vi "LV to DAT 1D.vi"(4 "append to file? (new file:F)":bool, 6 "wavenames (.Vx, etc)":string[](array[string]), 7 "filename":string, 8 "error in":errorcluster, 9 "Data":dbl[](array[numeric]), 10 "Comments":string, 11 "path":path) -> (0 "error out":errorcluster, 3 "new file path":path)   [LabVIEW 2016, in "LV to ITX.lvclass"]
uses:
  LV to ITX.lvclass
  Typedefs/Filetype--enum.ctl
  <vilib>/Utility/file.llb/Write Delimited Spreadsheet (string).vi
panel:
  out "appended array":string[][](array[string])
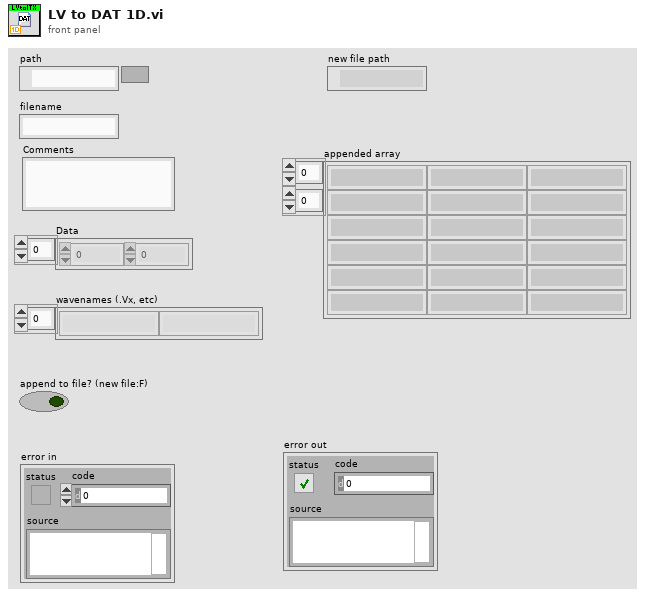
[diagram p1: front panel]
types:
  T1 = typedef "LV to ITX.lvclass/Filetype--enum.ctl" = enum16{"DAT", "ITX", "HDF5", "TDMS", "VI"}
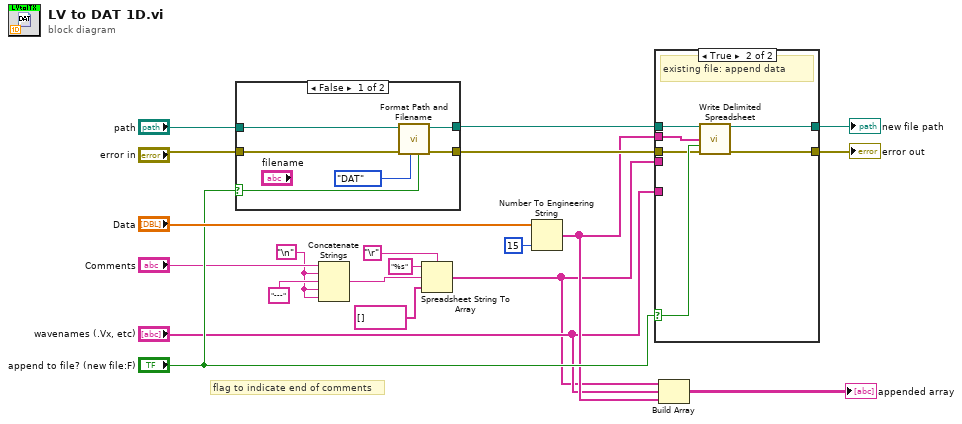
[diagram p0: block diagram]
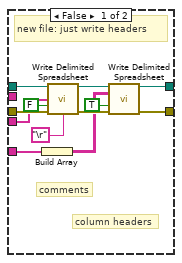
[diagram p3: hidden frame]
diagram:
  w6 = "\n"
  # "flag to indicate end of comments"
  n1 = case shown="False" "append to file? (new file:F)" {
    selector: "append to file? (new file:F)" -> [w22 _]
    tunnel: [w24 w28] -> w20
    tunnel: "path" -> [w25 w28]
    tunnel: "error in" -> [w26 w27]
    tunnel: [w23 w27] -> w14
    frame False {
      n2 = call "Format Path and Filename.vi"("append? (F)"=w22, "Type (TDMS)"=Filetype--enum."DAT", "error in"=w26, "path"=w25) -> ("error out"=w23:errorcluster, "path"=w24:path)  [unwired: 5 in, 1 out]
    }
    frame True {
    }
  }
  n3 = Concatenate Strings("Comments", w6, "---" ("string"), w6, w6) -> (w11:string)
  n4 = Spreadsheet String To Array(delimiter (Tab)="\r", format string="%s", spreadsheet string=w11, array type (2D Dbl)=string[] []) -> (array=w2:string[])
  n5 = Number To Engineering String(2:i16 15 ("precision (6)"), 4:"Data") -> (0:w4:string[])  [unwired: 2 out]
  n6 = case shown="True" "append to file? (new file:F)" {
    selector: "append to file? (new file:F)" -> [_ w45]
    tunnel: w2 -> [w33 _]
    tunnel: [w38 w42] -> w13
    tunnel: w4 -> [_ w44]
    tunnel: w20 -> [w40 w46]
    tunnel: w14 -> [w39 w43]
    tunnel: [w35 w41] -> w12
    tunnel: "wavenames (.Vx, etc)" -> [w32 _]
    frame False {
      # "column headers"
      # "comments"
      # "new file: just write headers"
      n7 = Build Array(w32) -> (w31:string[][])
      n8 = call-poly <vilib>:"Write Delimited Spreadsheet.vi"("file path (dialog if empty)"=w40, "1D data"=w33, "append to file? (new file:F)"=FALSE, "error in (no error)"=w39, "delimiter (\\t)"="\r") -> ("new file path (Not A Path if cancelled)"=w36:path, "error out"=w37:errorcluster)  [unwired: 9 in]
      n9 = call-poly <vilib>:"Write Delimited Spreadsheet.vi"("file path (dialog if empty)"=w36, "2D data"=w31, "append to file? (new file:F)"=TRUE, "error in (no error)"=w37) -> ("new file path (Not A Path if cancelled)"=w38:path, "error out"=w35:errorcluster)  [unwired: 10 in]
    }
    frame True {
      # "existing file: append data"
      n10 = call-poly <vilib>:"Write Delimited Spreadsheet.vi"("file path (dialog if empty)"=w46, "1D data"=w44, "append to file? (new file:F)"=w45, "error in (no error)"=w43) -> ("new file path (Not A Path if cancelled)"=w42:path, "error out"=w41:errorcluster)  [unwired: 10 in]
    }
  }
  "new file path" <- w13
  "error out" <- w12
  n11 = Build Array(w2, "wavenames (.Vx, etc)", w4) -> (→"appended array":string[][])
